vi "test_Create Instrument Addon.vi"(8 "error in (no error)":errorcluster, 11 "TestCase in":refnum<class "Instrument Addon Scripting API Custom Device Unit Tests.lvclass">) -> (0 "error out":errorcluster, 3 "TestCase out":refnum<class "Instrument Addon Scripting API Custom Device Unit Tests.lvclass">)   [LabVIEW 2018, in "Instrument Addon Scripting API Custom Device Unit Tests.lvclass"]
uses:
  Instrument Addon Scripting API Custom Device Unit Tests.lvclass
  Addon/Support Libraries/Protocols.lvlibp/TCP/TCP Settings.ctl
  Addon/Support Libraries/Protocols.lvlibp/TCP/TCP.lvclass
  D:/GitRepository/niveristand-instrument-addon-custom-device/Source/Addon/Support Libraries/Protocols.lvlibp/Protocol Parent/Protocol Parent.lvclass
  NationalInstruments.VeriStand.SystemDefinitionAPI
  Instrument Addon Scripting API Custom Device Unit Tests.lvclass/Instrument Addon Scripting API Custom Device Unit Tests.ctl
  Addon/Addon Shared/SubVIs/Constants.vi
  <vilib>/NI/NI VeriStand Advanced SysDef API/_SubVIs/SysDef.Search.GUID.vi
  <vilib>/addons/_JKI Toolkits/VI Tester/TestCase.llb/TestCase.lvclass
  Instrument Addon Scripting API Test Assets/Instrument Addon Scripting API Test Assets.lvclass
  APIs/Scripting API/Instrument Addon Scripting API.lvlib
  <vilib>/NI/NI VeriStand Advanced SysDef API/SysDef API/Advanced System Definition.lvlib
  Addon/Addon Shared/Instrument Addon Shared.lvlib
  C:/Program Files (x86)/National Instruments/LabVIEW 2018/vi.lib/addons/_JKI Toolkits/VI Tester/TestCase.llb/TestCase.lvclass
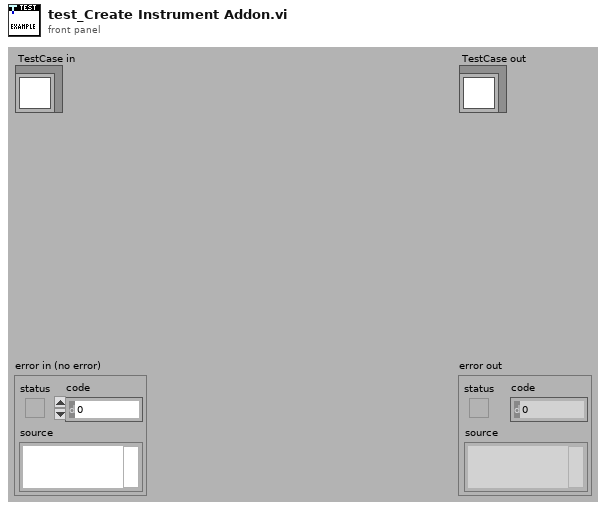
[diagram p1: front panel]
types:
  T1 = typedef "Protocols.lvlibp/TCP.lvclass/TCP Settings.ctl" = cluster{"IP Address":string, "Port":u16}
  T2 = typedef "Custom Device API.lvlib/Custom Device Item Ref.ctl" = u64
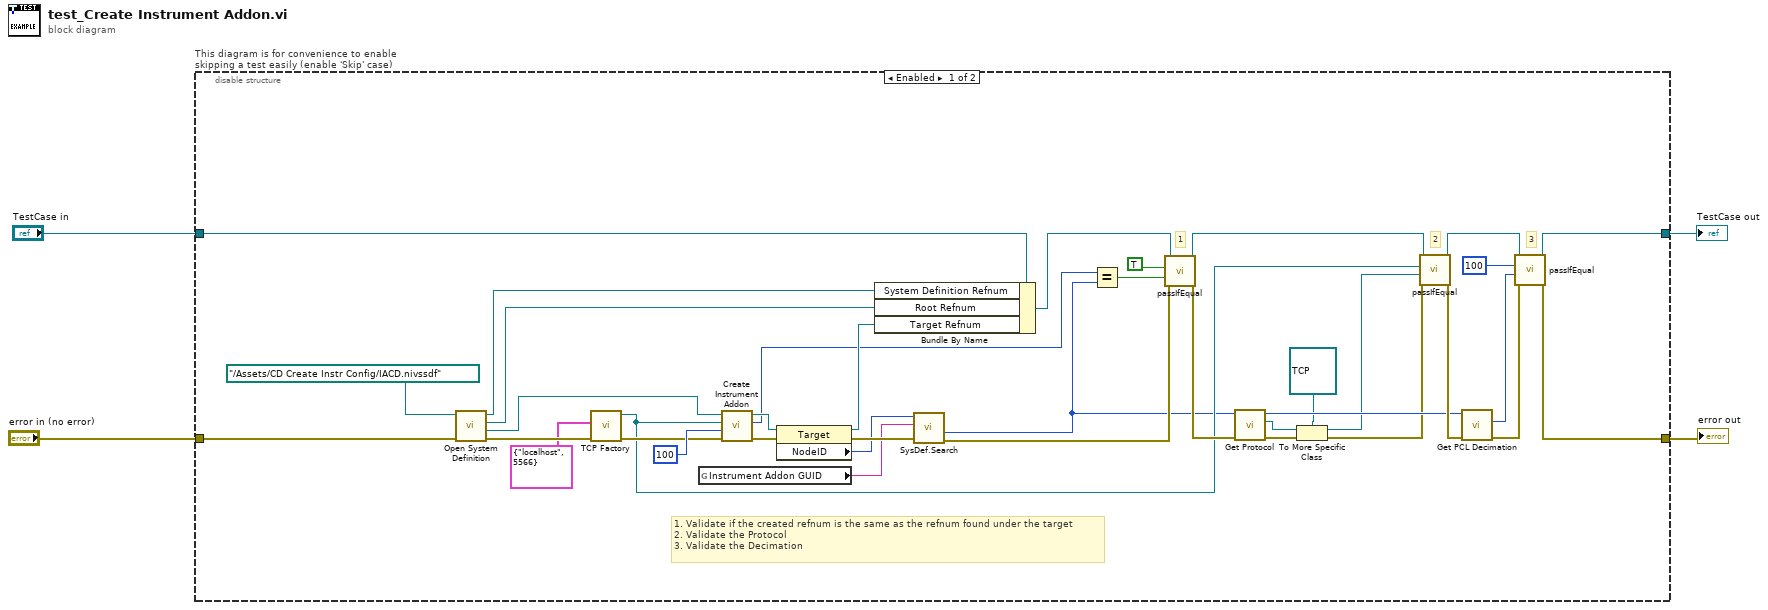
[diagram p0: block diagram]
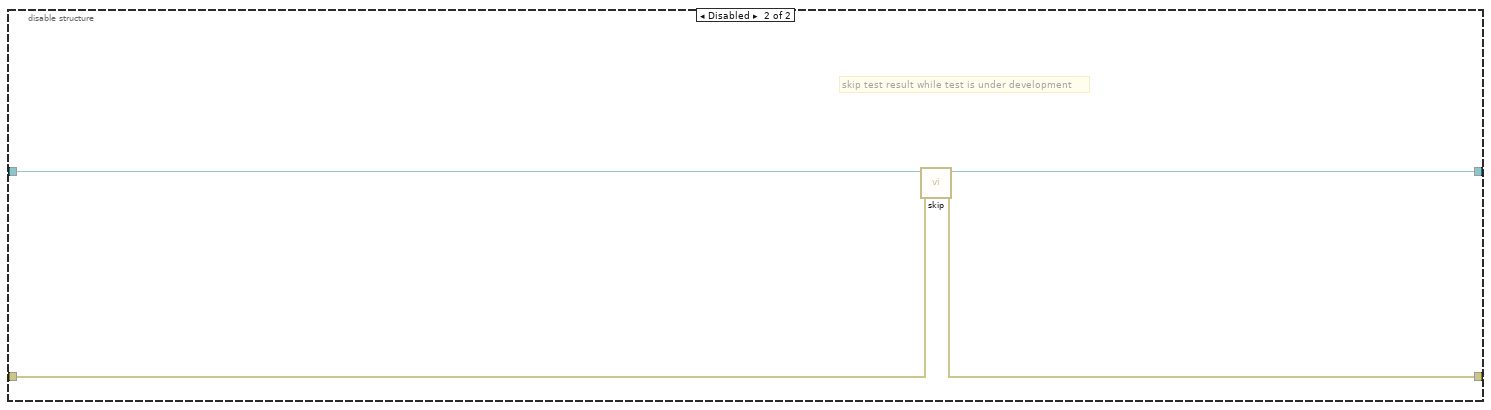
[diagram p2: hidden frame]
diagram:
  n1 = disable-structure "This diagram is for convenience to enable skipping a test easily (enable 'Skip' case)" shown="Enabled" {
    disable-tunnel: "TestCase in" -> [w39 w46]
    disable-tunnel: [w14 w44] -> w1
    disable-tunnel: [w15 w45] -> w3
    disable-tunnel: "error in (no error)" -> [w37 w43]
    frame Enabled {
      # "1. Validate if the created refnum is the same as the refnum found under the target\n2. Validate the Protocol\n3. Validate the Decimation"
      # "3"
      # "2"
      # "1"
      n2 = call "Open System Definition.vi"("error in (no error)"=w37, "System Definition File"=path "../Assets/CD Create Instr Config/IACD.nivssdf") -> ("error out"=w34:errorcluster, "Target Refnum"=w33:refnum<k24>, "Root Refnum"=w40:refnum<k24>, "System Definition Refnum"=w41:refnum<k24>)  [unwired: 6 in]
      n3 = call "TCP Factory.vi"("Error In"=w34, "TCP Settings"=T1 {"IP Address"="localhost", "Port"=5566}) -> ("Error Out"=w35:errorcluster, "TCP Out"=w23:refnum<class "TCP.lvclass">)  [unwired: 8 in]
      n4 = global read "Constants.vi" "Instrument Addon GUID"() -> (w27:string)
      n5 = call "Create Instrument Addon.vi"("Error In"=w35, "PCL Decimation"=u16 100, "Protocol In"=w23, "Target in"=w33) -> ("Error Out"=w30:errorcluster, "Instrument Addon Refnum"=w12:T2, "Target Out"=w31:refnum<k24>)  [unwired: 5 in]
      n6 = property class="Target"(reference=w31, error in=w30) -> (reference out=w25:refnum<k24>, error out=w29:errorcluster, "NodeID"=w26:u64)
      n7 = Bundle By Name(cluster=w39, "System Definition Refnum"=w41, "Root Refnum"=w40, "Target Refnum"=w25) -> (w38:refnum<class "Instrument Addon Scripting API Custom Device Unit Tests.lvclass">)
      n8 = call-poly <vilib>:"SysDef.Search.vi"("error in (no error)"=w29, "GUID"=w27, "nodeID"=w26) -> ("error out"=w28:errorcluster, "Value out"=w13:u64)  [unwired: 5 in, 2 out]
      n9 = Equal?(x=w12, y=w13) -> (x = y?=w11:bool)
      n10 = call-dynamic "passIfEqual.vi"("error in (no error)"=w28, "y"=w11, "x"=TRUE ("x = y?"), "TestCase in"=w38) -> ("error out"=w24:errorcluster, "TestCase out"=w22:refnum<class "Instrument Addon Scripting API Custom Device Unit Tests.lvclass">)  [unwired: 6 in]
      n11 = call "Get Protocol.vi"("Error In"=w24, "Instrument Addon Refnum In"=w13) -> ("Error Out"=w8:errorcluster, "Protocol"=w9:refnum<class "Protocol Parent.lvclass">, "Instrument Addon Refnum Out"=w20:T2)  [unwired: 7 in]
      n12 = To More Specific Class(target class=refnum<class "TCP.lvclass"> refnum ("Protocols.lvlibp:TCP.lvclass"), reference=w9, error in=w8) -> (specific class reference=w5:refnum<class "TCP.lvclass">, error out=w7:errorcluster)
      n13 = call-dynamic "passIfEqual.vi"("error in (no error)"=w7, "y"=w5, "x"=w23, "TestCase in"=w22) -> ("error out"=w21:errorcluster, "TestCase out"=w16:refnum<class "Instrument Addon Scripting API Custom Device Unit Tests.lvclass">)  [unwired: 6 in]
      n14 = call "Get PCL Decimation.vi"("Error In"=w21, "Instrument Addon Refnum In"=w20) -> ("Error Out"=w19:errorcluster, "PCL Decimation"=w18:u32)  [unwired: 7 in, 1 out]
      n15 = call-dynamic "passIfEqual.vi"("error in (no error)"=w19, "y"=w18, "x"=u32 100 ("PCL Decimation"), "TestCase in"=w16) -> ("error out"=w15:errorcluster, "TestCase out"=w14:refnum<class "Instrument Addon Scripting API Custom Device Unit Tests.lvclass">)  [unwired: 6 in]
    }
    frame Disabled {
      # "skip test result while test is under development"
      n16 = call <vilib>:"skip.vi"("error in (no error)"=w43, "TestCase in"=w46) -> ("error out"=w45:errorcluster, "TestCase out"=w44:refnum<class "Instrument Addon Scripting API Custom Device Unit Tests.lvclass">)  [unwired: 8 in]
    }
  }
  "error out" <- w3
  "TestCase out" <- w1
